vi "Process.vi"(8 "error in (no error)":errorcluster, 10 "Pound in":refnum<class "Pound.lvclass">, 11 "Qbus in":refnum<class "Qbus.lvclass">) -> (0 "error out":errorcluster)   [LabVIEW 2017, in "TrendAlarm.lvlib"]
uses:
  <vilib>/addons/InsightCM/Devices/Shared/Common/TrendAlarm/TrendAlarm.lvlib
  <vilib>/addons/Qbus/Qbus.lvclass
  <vilib>/NI/Software Watchdog/Pound/Pound.lvclass
  <vilib>/addons/InsightCM/Devices/Shared/Common/TrendAlarm/controls/config.ctl
  <vilib>/addons/InsightCM/Devices/Shared/Common/TrendAlarm/controls/TransitionCache.ctl
  <vilib>/addons/InsightCM/MessageBus/Base/controls/TrendAlarmTransition.ctl
  <vilib>/addons/TraceLogger/TraceLogger.lvlib
  <vilib>/NI/Software Watchdog/Watchdog/Watchdog.lvclass
  <vilib>/addons/InsightCM/Devices/Shared/Common/DataFlow/DataFlow.lvlib
  <vilib>/addons/InsightCM/Devices/Shared/Common/ServerComm/ServerComm.lvlib
  <vilib>/addons/InsightCM/Utilities/GlobalConfiguration/GlobalConfiguration.lvlib
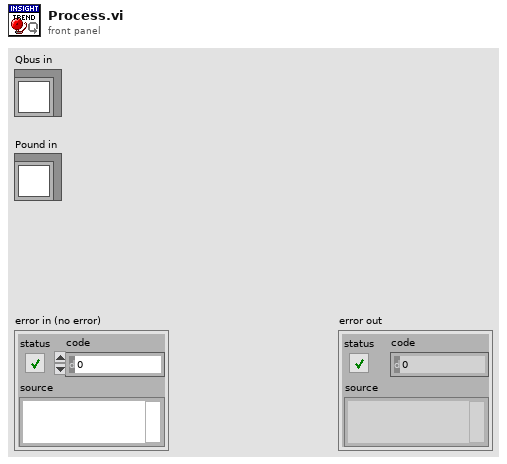
[diagram p1: front panel]
types:
  T1 = typedef "TrendAlarm.lvlib/config.ctl" = cluster{"Rules":variant, "Transitions":variant, "Online":bool, "ReceivedActive":bool, "DeviceName":string, "delayInitialized":bool}
  T2 = typedef "TrendAlarm.lvlib/TransitionCache.ctl" = cluster{"RuleId":string, "MaxSeverity":i32, "LastTransition":T3, "OnTime":timestamp, "OffTime":timestamp}
  T3 = typedef "TrendAlarmTransition.ctl" = cluster{"At":i64, "Severity":i32, "Value":dbl}
  T4 = typedef "ServerComm.lvlib/ConnectionStatus.ctl" = enum16{"Offline", "NotAuthorized", "Online"}
  T5 = typedef "Message.ctl" = cluster{"Header":T6, "Body":u8[]}
  T6 = typedef "MessageHeader.ctl" = cluster{"MessageName":string, "Timestamp":i64, "CorrelationId":string, "ContentType":string, "RoutingKey":string, "Properties":T7[]}
  T7 = typedef "KeyValuePair.ctl" = cluster{"Key":string, "Value":string}
  T8 = typedef "AlarmQueryActiveTrendInstancesResponseBody.ctl" = cluster{"ActiveAlarms":T9[], "Annotations":T10[], "TotalCount":i32}
  T9 = typedef "TrendAlarmInstance.ctl" = cluster{"Id":string, "RuleId":string, "Active":bool, "Acknowledged":bool, "AckAt":i64, "MaxSeverity":i32, "Transitions":T3[]}
  T10 = typedef "Annotation.ctl" = cluster{"Id":string}
  T11 = typedef "DeviceTrendAlarmUpdatedRoutedMessageBody.ctl" = cluster{"Updates":T12[]}
  T12 = typedef "DeviceTrendAlarmUpdate.ctl" = cluster{"RuleId":string, "Transition":T3, "MaxSeverity":i32}
  T13 = typedef "DataFlow.lvlib/Data.ctl" = cluster{"DataGroup":string, "Waveforms":T14, "Map":T15, "Type":T16}
  T14 = typedef "wfmSGL_DVR.ctl" = refnum<data-value>
  T15 = typedef "PointValueMap.lvlib/PointMap.ctl" = refnum<data-value>
  T16 = typedef "DataFlow.lvlib/Type.ctl" = enum16{"High Rate", "Low Rate", "Burst Mode"}
  T17 = typedef "DeviceTrendAlarmInactiveRoutedMessageBody.ctl" = cluster{"RuleId":string}
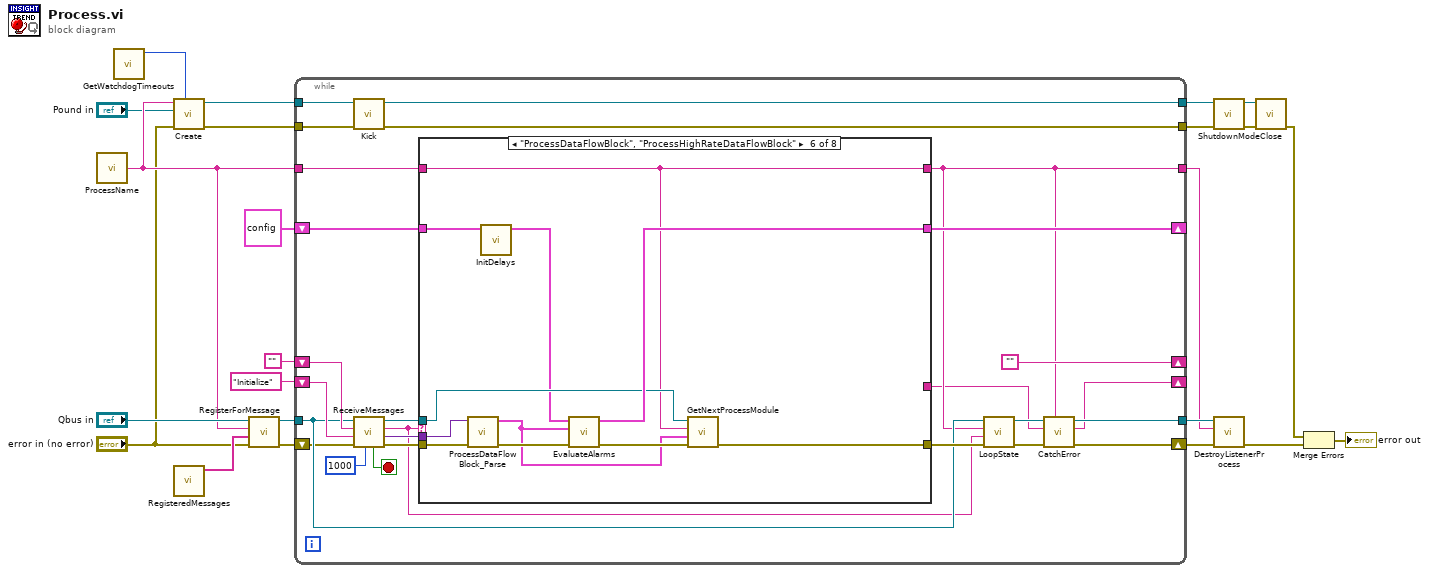
[diagram p0: block diagram]
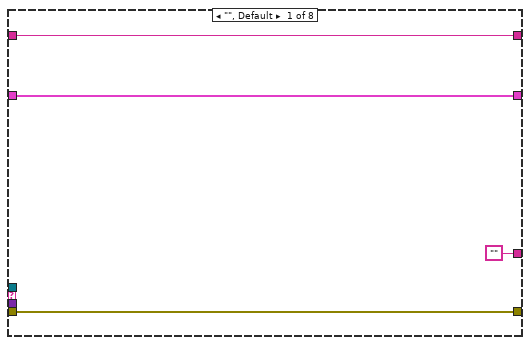
[diagram p2: hidden frame]
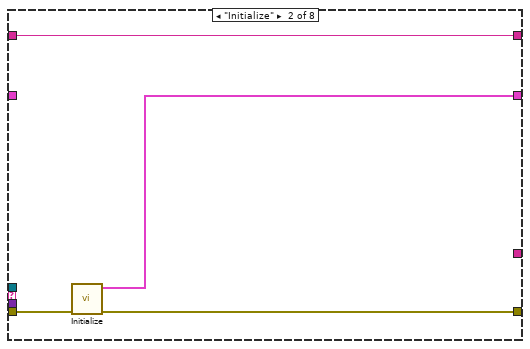
[diagram p3: hidden frame]
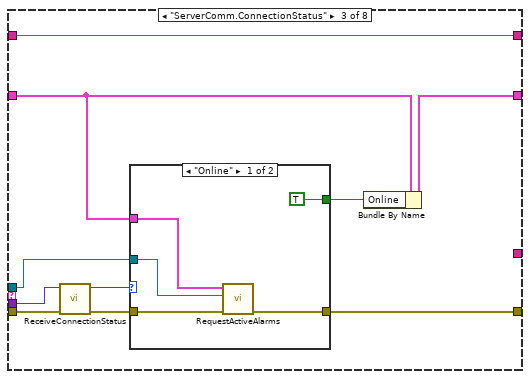
[diagram p4: hidden frame]
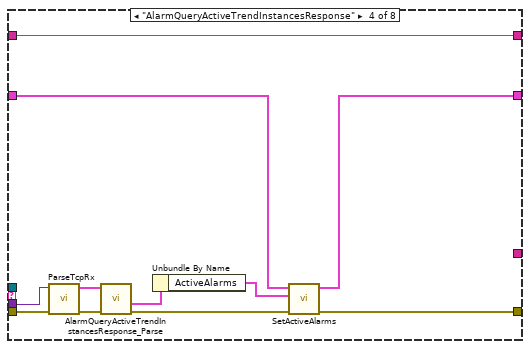
[diagram p6: hidden frame]
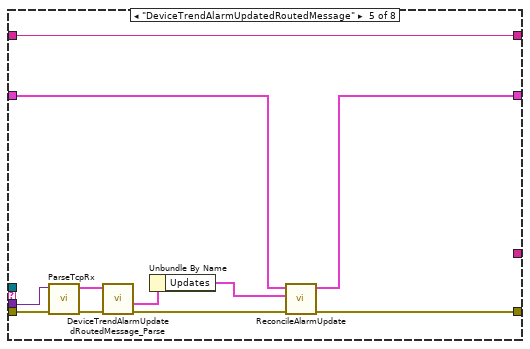
[diagram p7: hidden frame]
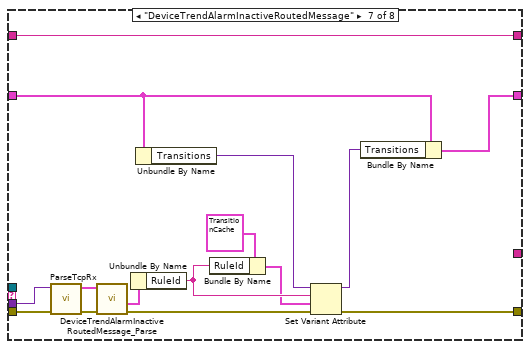
[diagram p8: hidden frame]
diagram:
  n1 = call <vilib>:"ProcessName.vi"() -> ("process name"=w13:string)  [unwired: 5 in]
  n2 = call <vilib>:"GetWatchdogTimeouts.vi"() -> ("software timeout"=w1:u32)  [unwired: 10 in, 1 out]
  n3 = call <vilib>:"Create.vi"("Execution Timeout (ms)"=w1, "error in (no error)"="error in (no error)", "Pound"="Pound in", "Name"=w13) -> ("error out"=w7:errorcluster, "Watchdog"=w12:refnum<data-value>)  [unwired: 6 in]
  n4 = call <vilib>:"RegisteredMessages.vi"() -> ("registered messages"=w14:string[])  [unwired: 11 in]
  n5 = call <vilib>:"RegisterForMessage.vi"("error in (no error)"="error in (no error)", "message names"=w14, "process name"=w13, "Qbus in"="Qbus in") -> ("error in (no error)"=w22:errorcluster, "Qbus out"=w21:refnum<class "Qbus.lvclass">)  [unwired: 6 in]
  n6 = while {
    shift-right: [""] -> _
    shift-left: "" -> [w48]
    tunnel: w21 -> [w36]
    tunnel: w13 -> [w26]
    tunnel: [w39] -> w19
    tunnel: [w25] -> w18
    shift-right: [w38] -> _
    shift-left: "Initialize" -> [w43]
    shift-right: [w41] -> _
    shift-left: T1 {"Rules"=variant(string ""), "Transitions"=variant, "Online"=FALSE, "ReceivedActive"=FALSE, "DeviceName"="", "delayInitialized"=FALSE} ("config") -> [w42]
    tunnel: w12 -> [w35]
    tunnel: [w34] -> w9
    tunnel: w7 -> [w33]
    tunnel: [w31] -> w6
    shift-right: [w40] -> w20
    shift-left: w22 -> [w32]
    stop <- w49 stop-if-true
    n7 = call <vilib>:"Kick.vi"("error in (no error)"=w33, "Watchdog"=w35) -> ("error out"=w31:errorcluster, "Watchdog"=w34:refnum<data-value>)  [unwired: 8 in]
    n8 = call <vilib>:"ReceiveMessages.vi"("Timeout(1000)"=1000 ("milliseconds to wait"), "error in (no error)"=w32, "priority action"=w43, "default action"=w48, "Qbus in"=w36) -> ("error out"=w47:errorcluster, "message value"=w44:variant, "action"=w30:string, "Qbus out"=w45:refnum<class "Qbus.lvclass">, "exit"=w49:bool)  [unwired: 2 in]
    n9 = case shown="\"ProcessDataFlowBlock\", \"ProcessHighRateDataFlowBlock\"" w30 {
      tunnel: w47 -> [w50 w56 w66 w83 w94 w105 w120 w124]
      tunnel: w45 -> [_ _ w59 _ _ w100 _ _]
      tunnel: [w50 w55 w58 w78 w88 w101 w109 w124] -> w37
      tunnel: w44 -> [_ _ w65 w82 w93 w106 w118 _]
      tunnel: w42 -> [w53 _ w61 w81 w87 w97 w115 w123]
      tunnel: [w53 w54 w63 w80 w86 w103 w114 w123] -> w41
      tunnel: [w52 w57 w67 w84 w95 w99 w121 w122] -> w25
      tunnel: w26 -> [w52 w57 w67 w84 w95 w99 w121 w122]
      tunnel: ["" _ _ _ _ _ _ _] -> w24
      frame "", Default {
      }
      frame "Initialize" {
        n10 = call <vilib>:"Initialize.vi"("error in (no error)"=w56) -> ("error out"=w55:errorcluster, "config"=w54:T1)  [unwired: 9 in]
      }
      frame "ServerComm.ConnectionStatus" {
        n11 = call <vilib>:"ReceiveConnectionStatus.vi"("error in (no error)"=w66, "body"=w65) -> ("error out"=w60:errorcluster, "status"=w64:T4)  [unwired: 6 in, 2 out]
        n12 = case shown="\"Online\"" w64 {
          tunnel: [TRUE _] -> w62
          tunnel: w61 -> [w70 _]
          tunnel: w60 -> [w71 w73]
          tunnel: w59 -> [w69 _]
          tunnel: [w68 w73] -> w58
          frame "Online" {
            n13 = call <vilib>:"RequestActiveAlarms.vi"("error in (no error)"=w71, "Qbus in"=w69, "config"=w70) -> ("error out"=w68:errorcluster)  [unwired: 8 in]
          }
          frame Default {
          }
        }
        n14 = Bundle By Name(cluster=w61, "Online"=w62) -> (w63:T1)
      }
      frame "AlarmQueryActiveTrendInstancesResponse" {
        n15 = call <vilib>:"ParseTcpRx.vi"("error in (no error)"=w83, "body"=w82) -> ("error out"=w76:errorcluster, "message"=w77:T5)  [unwired: 8 in]
        n16 = call <vilib>:"AlarmQueryActiveTrendInstancesResponse_Parse.vi"("error in (no error)"=w76, "Message"=w77) -> ("error out"=w75:errorcluster, "Body"=w74:T8)  [unwired: 6 in, 2 out]
        n17 = Unbundle By Name(w74) -> ("ActiveAlarms"=w79:T9[])
        n18 = call <vilib>:"SetActiveAlarms.vi"("error in (no error)"=w75, "ActiveAlarms"=w79, "config in"=w81) -> ("error out"=w78:errorcluster, "config out"=w80:T1)  [unwired: 7 in]
      }
      frame "DeviceTrendAlarmUpdatedRoutedMessage" {
        n19 = call <vilib>:"ParseTcpRx.vi"("error in (no error)"=w94, "body"=w93) -> ("error out"=w91:errorcluster, "message"=w92:T5)  [unwired: 8 in]
        n20 = call <vilib>:"DeviceTrendAlarmUpdatedRoutedMessage_Parse.vi"("error in (no error)"=w91, "Message"=w92) -> ("error out"=w89:errorcluster, "Body"=w90:T11)  [unwired: 6 in, 2 out]
        n21 = Unbundle By Name(w90) -> ("Updates"=w85:T12[])
        n22 = call <vilib>:"ReconcileAlarmUpdate.vi"("error in (no error)"=w89, "Updates"=w85, "config in"=w87) -> ("error out"=w88:errorcluster, "config out"=w86:T1)  [unwired: 7 in]
      }
      frame "ProcessDataFlowBlock", "ProcessHighRateDataFlowBlock" {
        n23 = call <vilib>:"ProcessDataFlowBlock_Parse.vi"("error in (no error)"=w105, "body"=w106) -> ("error out"=w104:errorcluster, "data"=w98:T13)  [unwired: 8 in]
        n24 = call <vilib>:"InitDelays.vi"("config in"=w97) -> ("config out"=w96:T1)  [unwired: 10 in]
        n25 = call <vilib>:"EvaluateAlarms.vi"("error in (no error)"=w104, "data"=w98, "config in"=w96) -> ("error out"=w102:errorcluster, "config out"=w103:T1)  [unwired: 7 in]
        n26 = call <vilib>:"GetNextProcessModule.vi"("error in (no error)"=w102, "data"=w98, "source"=w99, "Qbus in"=w100) -> ("error out"=w101:errorcluster)  [unwired: 6 in, 1 out]
      }
      frame "DeviceTrendAlarmInactiveRoutedMessage" {
        n27 = call <vilib>:"ParseTcpRx.vi"("error in (no error)"=w120, "body"=w118) -> ("error out"=w119:errorcluster, "message"=w117:T5)  [unwired: 8 in]
        n28 = call <vilib>:"DeviceTrendAlarmInactiveRoutedMessage_Parse.vi"("error in (no error)"=w119, "Message"=w117) -> ("error out"=w110:errorcluster, "Body"=w116:T17)  [unwired: 6 in, 2 out]
        n29 = Unbundle By Name(w116) -> ("RuleId"=w108:string)
        n30 = Unbundle By Name(w115) -> ("Transitions"=w113:variant)
        n31 = Bundle By Name(cluster=T2 {"RuleId"="", "MaxSeverity"=0, "LastTransition"={"At"=0, "Severity"=0, "Value"=0.0}, "OnTime"=timestamp(0 s since 1904-01-01), "OffTime"=timestamp(0 s since 1904-01-01)} ("cache out"), "RuleId"=w108) -> (w107:T2)
        n32 = Set Variant Attribute(Variant=w113, name=w108, value=w107, error in=w110) -> (Variant out=w112:variant, error out=w109:errorcluster)  [unwired: 1 out]
        n33 = Bundle By Name(cluster=w115, "Transitions"=w112) -> (w114:T1)
      }
      frame "Exit" {
      }
    }
    n34 = call <vilib>:"LoopState.vi"("error in (no error)"=w37, "loop action"=w30, "process name"=w25, "Qbus in"=w36) -> ("error out"=w28:errorcluster, "Qbus out"=w27:refnum<class "Qbus.lvclass">)  [unwired: 6 in]
    n35 = call <vilib>:"CatchError.vi"("source"=w25, "error in (no error)"=w28, "next action in"=w24, "Qbus in"=w27) -> ("error out"=w40:errorcluster, "next action out"=w38:string, "Qbus out"=w39:refnum<class "Qbus.lvclass">)  [unwired: 5 in]
  }
  n36 = call <vilib>:"ShutdownMode.vi"("error in (no error)"=w6, "Watchdog"=w9) -> ("error out"=w8:errorcluster, "Watchdog"=w10:refnum<data-value>)  [unwired: 8 in]
  n37 = call <vilib>:"DestroyListenerProcess.vi"("error in (no error)"=w20, "process name"=w18, "Qbus in"=w19) -> ("error in (no error)"=w5:errorcluster)  [unwired: 7 in, 1 out]
  n38 = call <vilib>:"Close.vi"("error in (no error)"=w8, "Watchdog"=w10) -> ("error out"=w4:errorcluster)  [unwired: 9 in]
  n39 = Merge Errors(w4, w5) -> (→"error out":errorcluster)
